vi "loop-timer.vi"(11 "loop-time-in":u32) -> (1 "Loop Time (mS)":u32, 3 "loop-time-out":u32)   [LabVIEW 2024]
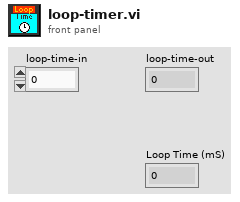
[diagram p1: front panel]
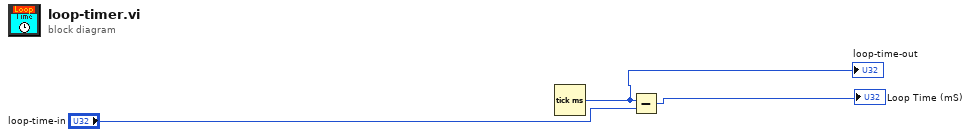
[diagram p0: block diagram]
diagram:
  n1 = Tick Count (ms)() -> (millisecond timer value=w2:u32)
  "loop-time-out" <- w2
  n2 = Subtract(x=w2, y="loop-time-in") -> (x-y=→"Loop Time (mS)":u32)
